vi "analog_read.vi"(8 "error in (no error)":errorcluster, 9 "Pin":u8=4 min=4 max=40, 11 "VISA resource name":refnum<visa-resource-name>) -> (0 "error out":errorcluster, 1 "Analog read":u16, 3 "VISA resource name out":refnum<visa-resource-name>)   [LabVIEW 2025]
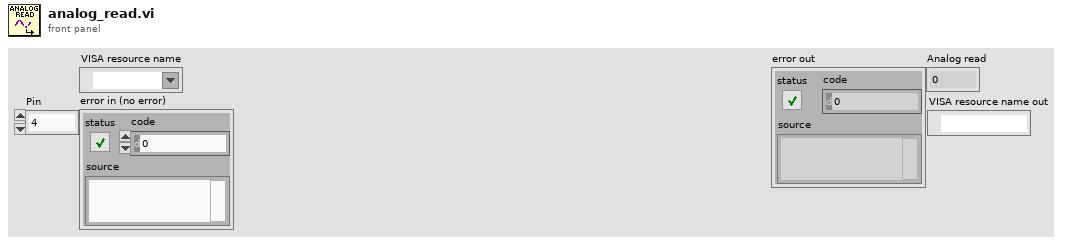
[diagram p1: front panel]
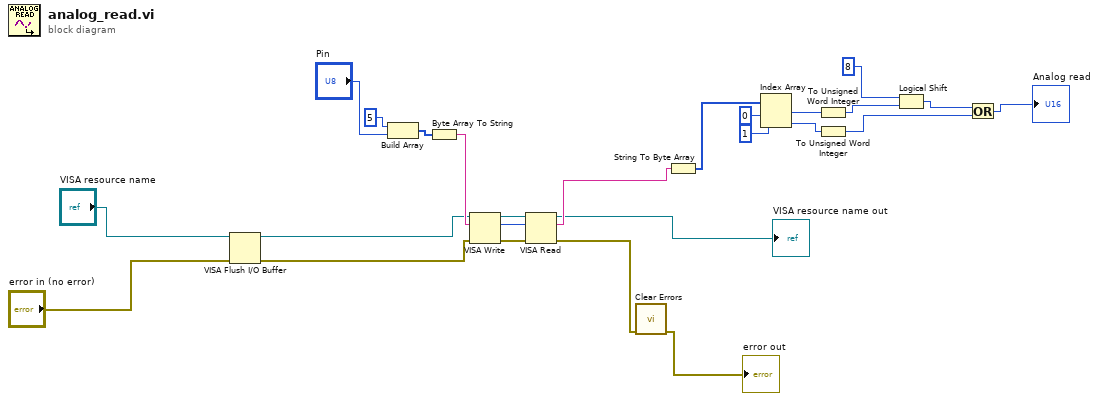
[diagram p0: block diagram]
diagram:
  n1 = VISA Flush I/O Buffer(VISA resource name="VISA resource name", error in (no error)="error in (no error)") -> (VISA resource name out=w18:refnum<visa-resource-name>, error out=w17:errorcluster)  [unwired: 1 in]
  n2 = Build Array(u8 5, "Pin") -> (w21:u8[])
  n3 = Byte Array To String(unsigned byte array=w21) -> (string=w25:string)
  n4 = VISA Write(VISA resource name=w18, write buffer=w25, error in (no error)=w17) -> (VISA resource name out=w23:refnum<visa-resource-name>, return count=w19:u32, error out=w24:errorcluster)
  n5 = VISA Read(VISA resource name=w23, byte count=w19, error in (no error)=w24) -> (VISA resource name out=→"VISA resource name out":refnum<visa-resource-name>, read buffer=w16:string, error out=w1:errorcluster)  [unwired: 1 out]
  n6 = call <vilib>:"Clear Errors.vi"("error in (no error)"=w1) -> ("error out"=→"error out":errorcluster)  [unwired: 5 in, 1 out]
  n7 = String To Byte Array(string=w16) -> (unsigned byte array=w15:u8[])
  n8 = Index Array(array=w15, index #1=0 ("index"), index #2=1 ("index")) -> (element #1=w8:u8, element #2=w9:u8)
  n9 = To Unsigned Word Integer(number=w8) -> (unsigned 16bit integer=w7:u16)
  n10 = To Unsigned Word Integer(number=w9) -> (unsigned 16bit integer=w6:u16)
  n11 = Logical Shift(y=8, x=w7) -> (x << y=w12:u16)
  n12 = Or(x=w12, y=w6) -> (x .or. y?=→"Analog read":u16)
